vi "Initialise.vi"(8 "error in (no error)":errorcluster, 10 "Message in":refnum<class "InitialiseMessage.lvclass">, 11 "ImageStack in":refnum<class "ImageStack.lvclass">) -> (0 "error out":errorcluster, 3 "ImageStack out":refnum<class "ImageStack.lvclass">)   [LabVIEW 2012, in "ImageStack.lvclass"]
doc: "This method is called when an initialise message is received. It mainly initialises the RabbitMQ connectivity. \n\nOverride this method when your component needs special initialisation (e.g. of software or hardware resources). In that case, don't forget to call the parent for proper implementation. If your component owns subcomponents, they count as resources, so you have to initialise them by calling their own initialise functions"
uses:
  ImageStack.lvclass
  <vilib>/Distrio/Murmex/InitialiseMessage/InitialiseMessage.lvclass
  <vilib>/Distrio/Murmex/Murmex/Murmex.lvclass
  <vilib>/Distrio/Murmex/GenericMessage/GenericMessage.lvclass
  ImageStack.lvclass/ImageStack.ctl
  <vilib>/Distrio/Murmex/Murmex/update_cluster.ctl
  <vilib>/Distrio/Murmex/Message/Add or replace parameter.vi
panel:
  # "This method is called when the INTIALISE\ntrigger is sent. \n\nOverride this method when your component needs to\nrespond to this trigger. \n\nCall parent for proper implementation"
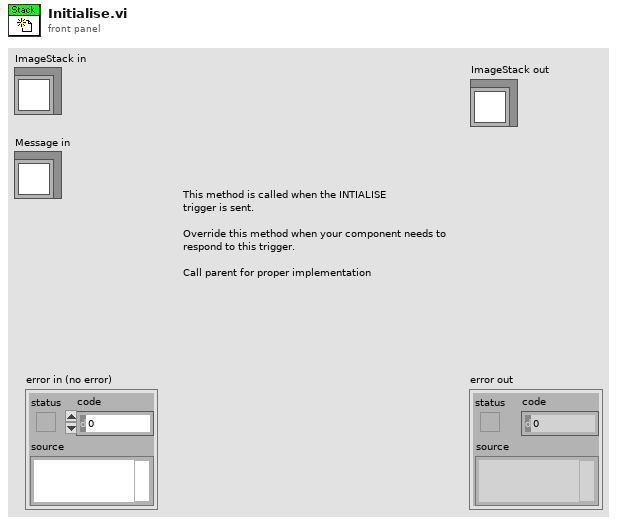
[diagram p1: front panel]
types:
  T1 = typedef "Murmex.lvlib/Murmex.lvclass/update_cluster.ctl" = cluster{"target ID":string, "key chains":string[], "values":variant[]}
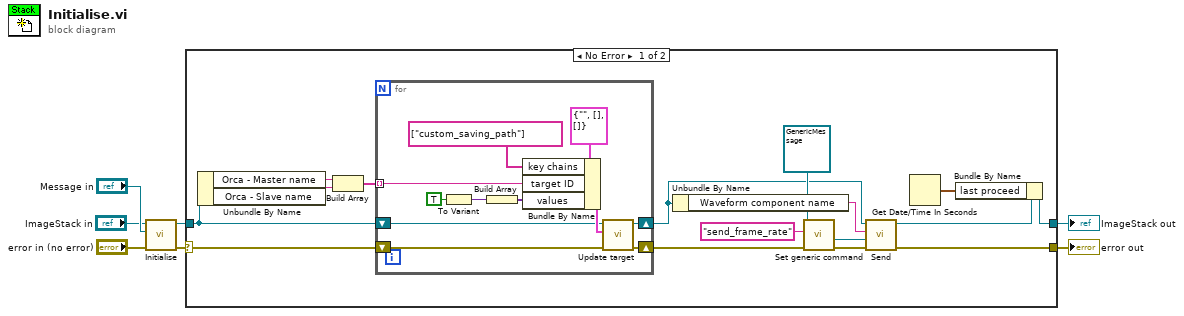
[diagram p0: block diagram]
diagram:
  n1 = call-parent "Initialise.vi"("error in (no error)"="error in (no error)", "Message in"="Message in", "Murmex in"="ImageStack in") -> ("error out"=w4:errorcluster, "Murmex out"=w1:refnum<class "ImageStack.lvclass">)  [unwired: 7 in]
  n2 = case shown="No Error" w4 {
    selector: w4 -> [w14 w36]
    tunnel: [w19 w36] -> w3
    tunnel: [w16 w35] -> w2
    tunnel: w1 -> [w11 w35]
    frame No Error {
      n3 = Unbundle By Name(w11) -> ("Orca - Master name"=w9:string, "Orca - Slave name"=w8:string)
      n4 = Build Array(w9, w8) -> (w10:string[])
      n5 = for {
        tunnel: w10 -> [w24] mode=indexing
        shift-right: [w26] -> w13
        shift-left: w11 -> [w25]
        shift-right: [w28] -> w21
        shift-left: w14 -> [w27]
        n6 = To Variant(anything=TRUE) -> (Variant=w30:variant)
        n7 = Build Array(w30) -> (w29:variant[])
        n8 = Bundle By Name(cluster=T1 {"target ID"="", "key chains"=[], "values"=[]} ("update cluster"), "key chains"=string[] ["custom_saving_path"], "target ID"=w24, "values"=w29) -> (w33:T1)
        n9 = call <vilib>:"Update target.vi"("error in (no error)"=w27, "update cluster"=w33, "MurmexBase in"=w25) -> ("error out"=w28:errorcluster, "MurmexBase out"=w26:refnum<class "ImageStack.lvclass">)  [unwired: 7 in]
      }
      n10 = Unbundle By Name(w13) -> ("Waveform component name"=w12:string)
      n11 = call <vilib>:"Set generic command.vi"("error in (no error)"=w21, "generic command"="send_frame_rate", "GenericMessage in"=refnum<class "GenericMessage.lvclass"> refnum ("Distrio Murmex 1.1:GenericMessage")) -> ("error out"=w20:errorcluster, "GenericMessage out"=w18:refnum<class "GenericMessage.lvclass">)  [unwired: 7 in]
      n12 = call <vilib>:"Send.vi"("error in (no error)"=w20, "Message"=w18, "recipient"=w12, "Murmex in"=w13) -> ("error out"=w19:errorcluster, "Murmex out"=w17:refnum<class "ImageStack.lvclass">)  [unwired: 6 in]
      n13 = Get Date/Time In Seconds() -> (seconds since 1Jan1904=w15:timestamp)
      n14 = Bundle By Name(cluster=w17, "last proceed"=w15) -> (w16:refnum<class "ImageStack.lvclass">)
    }
    frame Error {
    }
  }
  "error out" <- w3
  "ImageStack out" <- w2
